vi "niHWS Set Wfm String Attribute.vi"(8 "error in (no error)":errorcluster, 9 "attribute value":string, 10 "attribute ID":T1 items=["Note"=0, "X Axis Label"=1, "Y Axis Label"=2, "X Axis Units"=3, "Y Axis Units"=4, "Valid Signals"=6, "Timestamp"=7], 11 "waveform reference in":u32) -> (0 "error out":errorcluster, 3 "waveform reference out":u32)   [LabVIEW 2011]
doc: "Sets the value of text attributes that apply to the waveform specified by the waveform reference."
uses:
  niHWS Set Wfm String Attribute ID.ctl
  nihwsu.dll
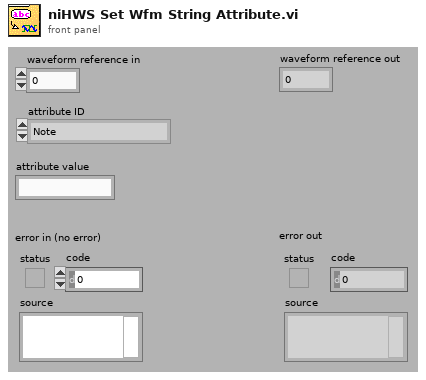
[diagram p1: front panel]
types:
  T1 = typedef "niHWS Set Wfm String Attribute ID.ctl" = u32
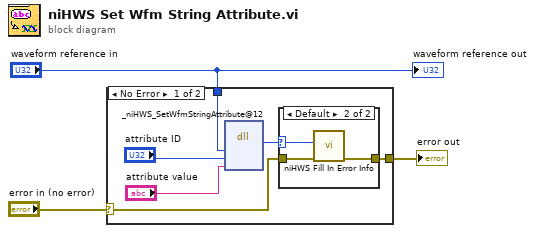
[diagram p0: block diagram]
diagram:
  n1 = case shown="No Error" "error in (no error)" {
    selector: "error in (no error)" -> [w6 w14]
    tunnel: [w7 w14] -> w2
    tunnel: "waveform reference in" -> [w8 _]
    frame No Error {
      n2 = dll-call lib="nihwsu.dll" fn="_niHWS_SetWfmStringAttribute@12"("wfmReference"=w8, "attributeID"="attribute ID", "attributeVal"="attribute value") -> (w5:i32)  [unwired: 6 in, 2 out]
      n3 = case shown="Default" w5 {
        selector: w5 -> [_ w11]
        tunnel: [w10 w12] -> w7
        tunnel: w6 -> [w10 w13]
        frame 0 {
        }
        frame Default {
          n4 = call "niHWS Fill In Error Info.vi"("error in (no error)"=w13, "status code"=w11) -> ("error out"=w12:errorcluster)  [unwired: 9 in]
        }
      }
    }
    frame Error {
    }
  }
  "error out" <- w2
  "waveform reference out" <- "waveform reference in"
